vi "Integrator.vi"   [LabVIEW 2020, in "NI_AdvCtrl_continuous linear.lvlib"]
doc: "LabVIEW no longer supports this VI. You can obtain similar functionality by installing the LabVIEW Simulation Module.\n\nIntegrates a continuous input signal. The integration process is based on Euler method. dt must be positive."
uses:
  <vilib>/addons/control/advanced/NI_AdvCtrl_continuous linear.lvlib
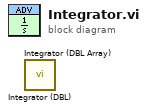
[diagram p0: block diagram]
diagram:
  n1 = call <vilib>:"Integrator (DBL).vi"() -> ()  [unwired: 5 in, 1 out]
  n2 = call <vilib>:"Integrator (DBL Array).vi"() -> ()  [unwired: 5 in, 1 out]
